vi "Main.vi"(8 "error in":errorcluster, 11 "New Worker in":refnum<class "Manager Worker.lvclass">) -> (0 "error out":errorcluster, 3 "New Worker out":refnum<class "Manager Worker.lvclass">)   [LabVIEW 2018, in "Manager Worker.lvclass"]
doc: "The Queued Message Handler of a Worker."
uses:
  Manager Worker.lvclass
  D:/Program Files (x86)/National Instruments/LabVIEW 2018/vi.lib/addons/_Workers/Library/Classes/Worker/Worker.lvclass
  Manager Worker.lvclass/Manager Worker.ctl
  <vilib>/addons/_Workers/Library/Classes/Worker/Worker.lvclass/Worker.ctl
  Initialization Data.ctl
  ChartView Worker/ChartView Worker.lvclass
  Config Worker/Config Worker.lvclass
  User Worker/User Worker.lvclass
  Comm Worker/Comm Worker.lvclass
  <vilib>/addons/_Workers/Library/Classes/Message/Enqueue Message to Queue.vi
  <vilib>/addons/_Workers/Library/Classes/Worker/Worker.lvclass
  <vilib>/addons/_Workers/Library/Classes/Message/Message.lvclass
  D:/Program Files (x86)/National Instruments/LabVIEW 2018/vi.lib/addons/_Workers/Library/Classes/Workers Object/Workers Object.lvclass
panel:
  in  "ButtonMenu":enum32{"ChartView", "Config", "User"}(radio)
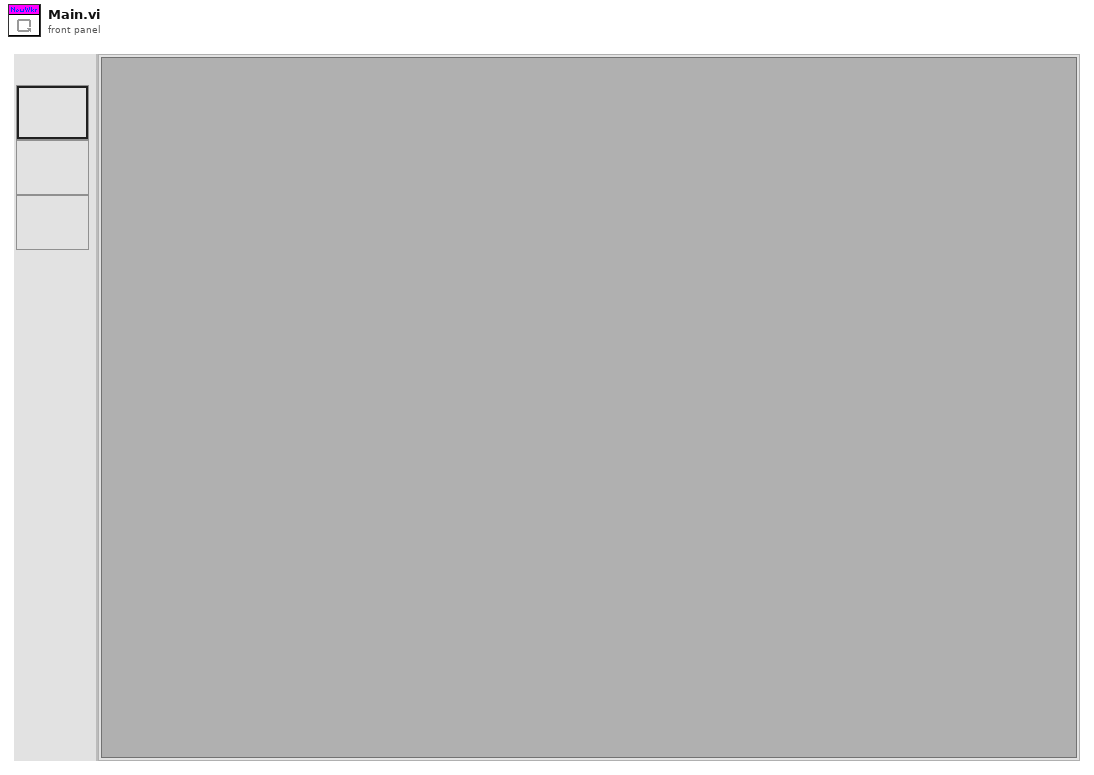
[diagram p1: front panel]
types:
  T1 = typedef "Manager Worker.lvclass/Initialization Data.ctl" = cluster{"String":string}
  T2 = typedef "Workers.lvlib/Case Label.ctl" = string
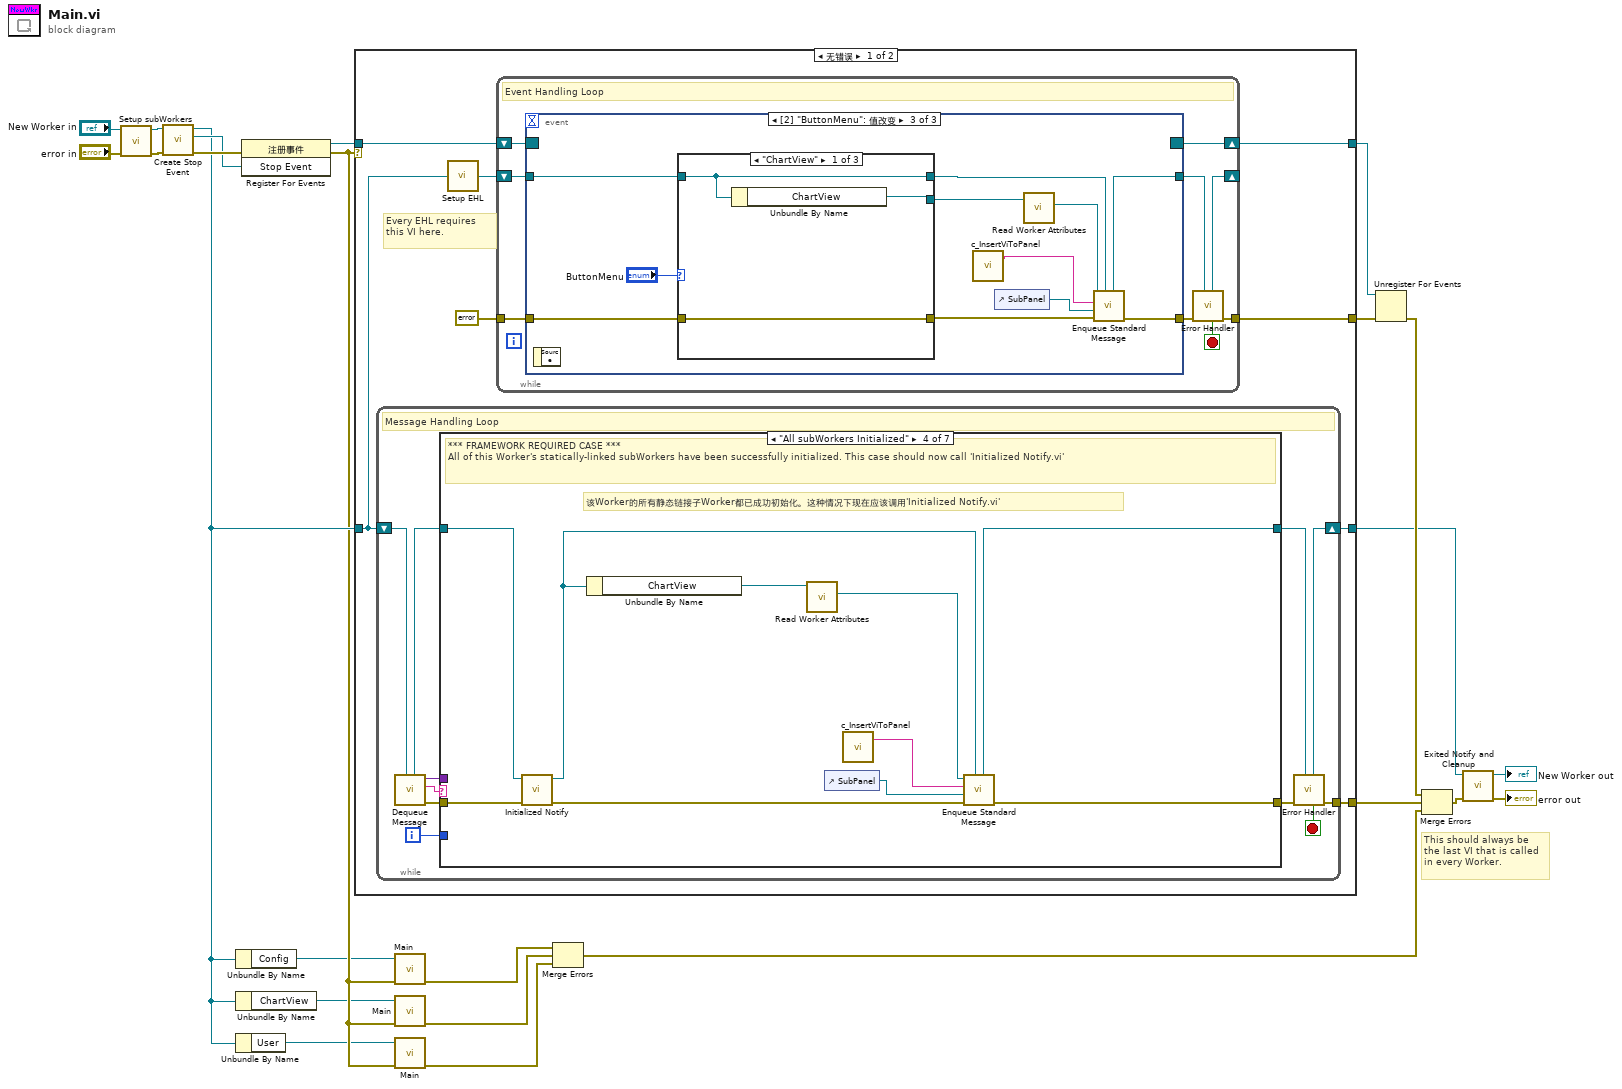
[diagram p0: block diagram]
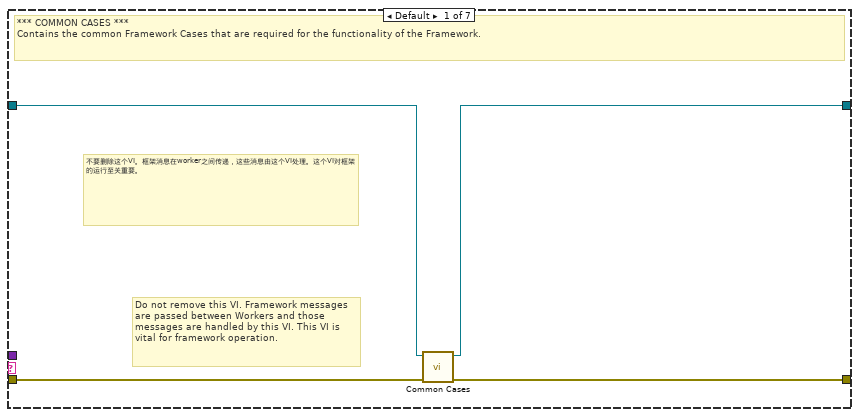
[diagram p2: hidden frame]
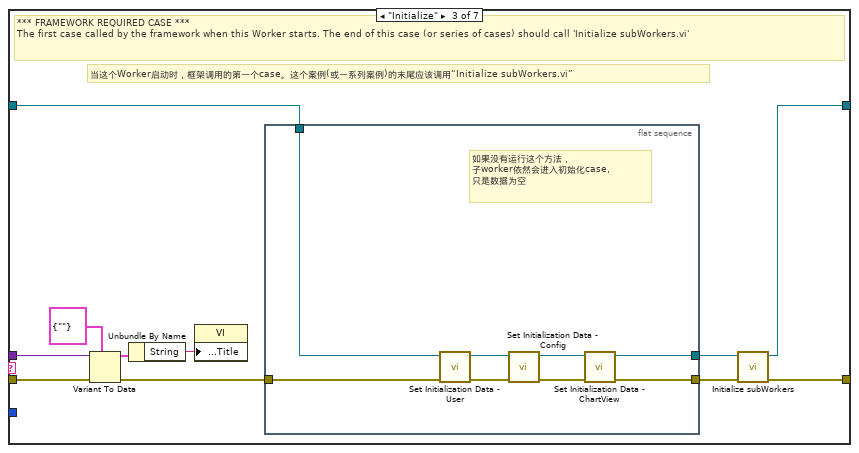
[diagram p4: hidden frame]
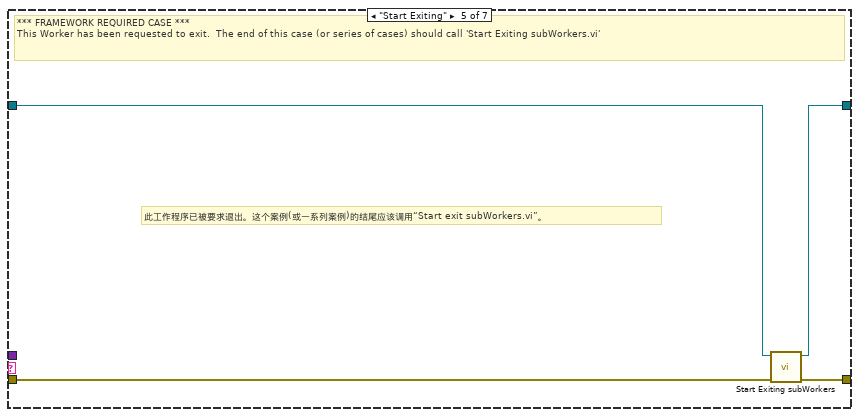
[diagram p5: hidden frame]
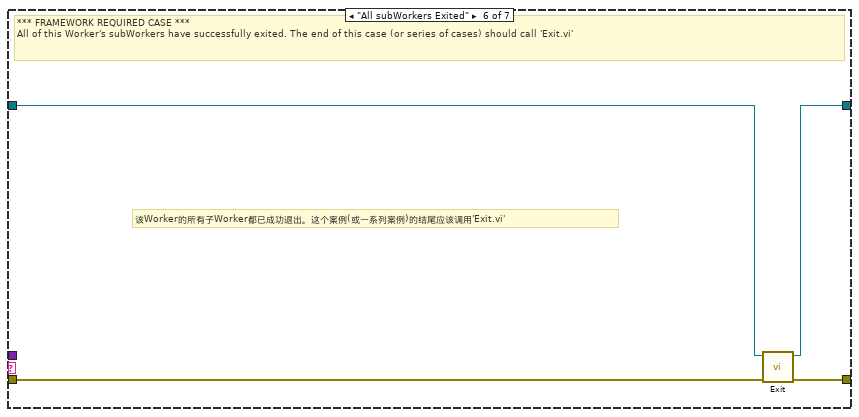
[diagram p6: hidden frame]
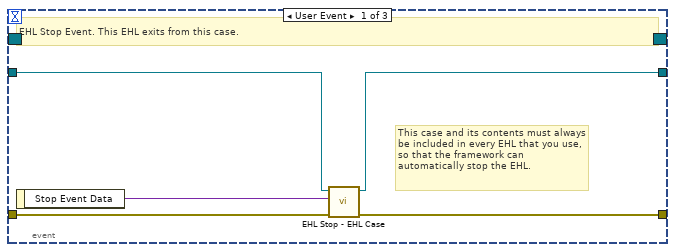
[diagram p8: hidden frame]
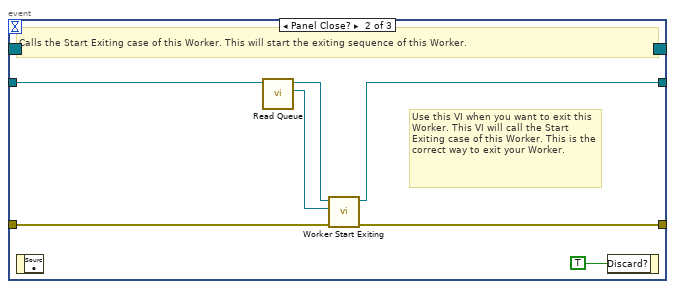
[diagram p9: hidden frame]
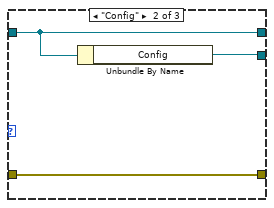
[diagram p10: hidden frame]
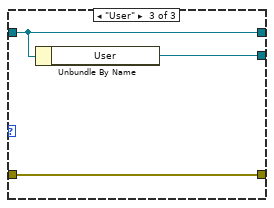
[diagram p11: hidden frame]
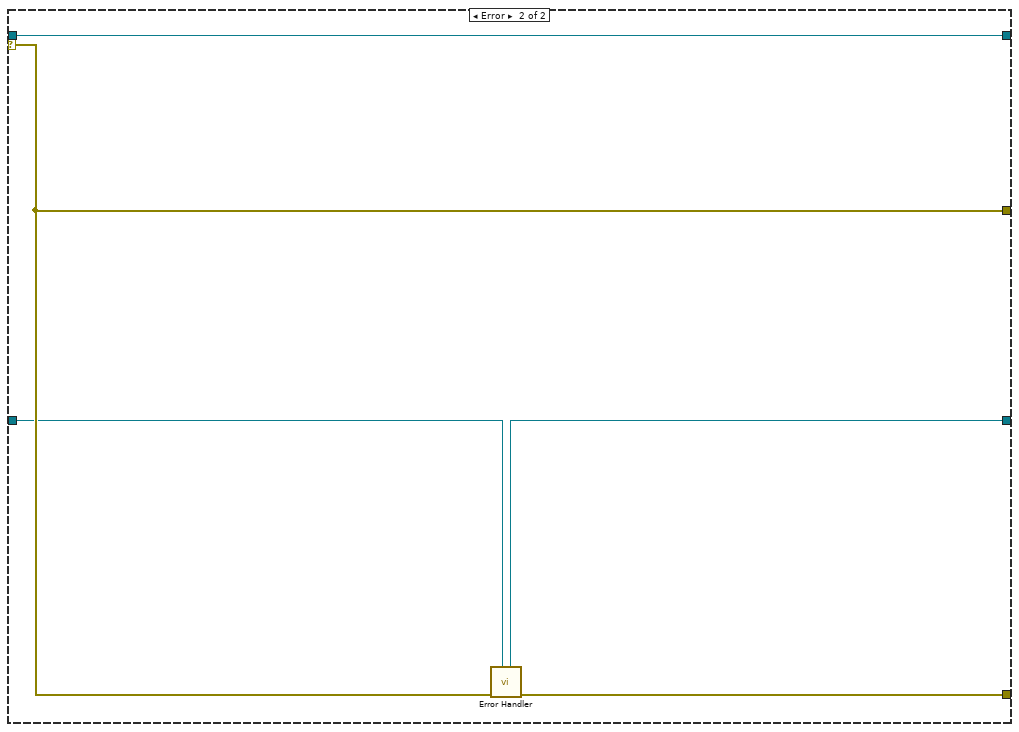
[diagram p12: hidden frame]
diagram:
  # "This should always be the last VI that is called in every Worker."
  n1 = call "Setup subWorkers.vi"("error in"="error in", "Manager Worker in"="New Worker in") -> ("error out"=w10:errorcluster, "Manager Worker out"=w8:refnum<class "Manager Worker.lvclass">)  [unwired: 8 in]
  n2 = call-dynamic "Create Stop Event.vi"("error in"=w10, "Worker"=w8) -> ("error out"=w19:errorcluster, "Stop Event"=w16:refnum<user-event>, "Worker out"=w13:refnum<class "Manager Worker.lvclass">)  [unwired: 7 in]
  n3 = Unbundle By Name(w13) -> ("Config"=w5:refnum<class "Config Worker.lvclass">)
  n4 = Unbundle By Name(w13) -> ("ChartView"=w3:refnum<class "ChartView Worker.lvclass">)
  n5 = Unbundle By Name(w13) -> ("User"=w1:refnum<class "User Worker.lvclass">)
  n6 = register-events(error in=w19, w16) -> (reference out=w18:refnum<event-registration>, error out=w11:errorcluster)  [unwired: 1 in]
  n7 = case shown="无错误" w11 {
    tunnel: w13 -> [w27 w131]
    tunnel: [w25 w132] -> w17
    tunnel: w18 -> [w32 w133]
    tunnel: [w29 w134] -> w23
    tunnel: [w31 w133] -> w22
    tunnel: [w26 w130] -> w20
    selector: w11 -> [_ w134]
    frame No Error {
      # "Every EHL requires\nthis VI here."
      n8 = while {
        shift-right: [w41] -> w26
        shift-left: w27 -> [w43]
        tunnel: [w42] -> w25
        i -> [w33]
        stop <- w34 stop-if-true
        # "Message Handling Loop"
        n9 = call-dynamic "Dequeue Message.vi"("Worker"=w43) -> ("error out"=w40:errorcluster, "Case out"=w35:string, "Data out"=w36:variant, "Worker out"=w38:refnum<class "Manager Worker.lvclass">)  [unwired: 6 in, 1 out]
        n10 = case "Worker MHL Case Structure (DO NOT CHANGE LABEL NAME)" shown="\"All subWorkers Initialized\"" w35 {
          tunnel: w40 -> [w47 w48 w58 w77 w79 w86 w87]
          tunnel: [w46 w48 w60 w75 w82 w85 w87] -> w39
          tunnel: w38 -> [w45 w49 w57 w78 w80 w84 w88]
          tunnel: [w44 w49 w59 w74 w81 w83 w88] -> w37
          tunnel: w36 -> [_ _ w56 _ _ _ _]
          tunnel: w33 -> [_ _ _ _ _ _ _]
          frame Default {
            # "不要删除这个VI。框架消息在worker之间传递，这些消息由这个VI处理。这个VI对框架的运行至关重要。"
            # "Do not remove this VI. Framework messages are passed between Workers and those messages are handled by this VI. This VI is vital for framework operation."
            # "*** COMMON CASES ***\nContains the common Framework Cases that are required for the functionality of the Framework."
            n11 = call-dynamic "Common Cases.vi"("error in"=w47, "Worker in"=w45) -> ("error out"=w46:errorcluster, "Worker out"=w44:refnum<class "Manager Worker.lvclass">)  [unwired: 8 in]
          }
          frame "------ FRAMEWORK REQUIRED CASES ------" {
            # "\"All subWorkers Exited\""
            # "\"Start Exiting\""
            # "\"All subWorkers Initialized\""
            # "\"Initialize\""
            # "启动机制。\n启动后会进入\"Initialize\" 分支，然后初始化下一层work.\n如果没有下一层work，则很快进入\"All subWorkers Initialized\" 分支。\n如果有下一层分支，则一层层的向下层初始化。然后又最底层的worker一层层向上发送 \"All subWorkers Initialized\" ，发送初始化完成通知。\n\n退出机制\n上层Worker进入\"Start Exiting\" 分支，向下一层发送 start Exiting Subworker。\n如果~~~\n如果有~~~\n与启动机制类似。"
            # "Start of Framework Required Cases"
          }
          frame "Initialize" {
            # "当这个Worker启动时，框架调用的第一个case。这个案例(或一系列案例)的末尾应该调用“Initialize subWorkers.vi”"
            # "*** FRAMEWORK REQUIRED CASE ***\nThe first case called by the framework when this Worker starts. The end of this case (or series of cases) should call 'Initialize subWorkers.vi'"
            n12 = Variant To Data(error in=w58, type=T1 {"String"=""} ("Initialization Data"), Variant=w56) -> (data=w54:T1, error out=w52:errorcluster)
            n13 = Unbundle By Name(w54) -> ("String"=w50:string)
            n14 = property class="VI"("Front Panel.Title"=w50) -> ()  [unwired: 2 in, 2 out]
            n15 = flat-sequence {
              tunnel: w57 -> [w68]
              tunnel: [w62] -> w53
              tunnel: w52 -> [w67]
              tunnel: [w61] -> w51
              frame #0 {
                # "如果没有运行这个方法，\n子worker依然会进入初始化case,\n只是数据为空"
                n16 = call "Set Initialization Data - User.vi"("error in"=w67, "Manager Worker in"=w68) -> ("error out"=w65:errorcluster, "Manager Worker out"=w66:refnum<class "Manager Worker.lvclass">)  [unwired: 8 in]
                n17 = call "Set Initialization Data - Config.vi"("error in"=w65, "Manager Worker in"=w66) -> ("error out"=w63:errorcluster, "Manager Worker out"=w64:refnum<class "Manager Worker.lvclass">)  [unwired: 8 in]
                n18 = call "Set Initialization Data - ChartView.vi"("error in"=w63, "Manager Worker in"=w64) -> ("error out"=w61:errorcluster, "Manager Worker out"=w62:refnum<class "Manager Worker.lvclass">)  [unwired: 8 in]
              }
            }
            n19 = call-dynamic "Initialize subWorkers.vi"("error in"=w51, "Worker"=w53) -> ("error out"=w60:errorcluster, "dup Worker out"=w59:refnum<class "Manager Worker.lvclass">)  [unwired: 8 in]
          }
          frame "All subWorkers Initialized" {
            # "该Worker的所有静态链接子Worker都已成功初始化。这种情况下现在应该调用'Initialized Notify.vi'"
            # "*** FRAMEWORK REQUIRED CASE ***\nAll of this Worker's statically-linked subWorkers have been successfully initialized. This case should now call 'Initialized Notify.vi'"
            n20 = call-dynamic "Initialized Notify.vi"("error in"=w77, "Worker"=w78) -> ("error out"=w76:errorcluster, "dup Worker out"=w72:refnum<class "Manager Worker.lvclass">)  [unwired: 8 in]
            n21 = Unbundle By Name(w72) -> ("ChartView"=w71:refnum<class "ChartView Worker.lvclass">)
            n22 = call-poly <vilib>:"Read Worker Attributes.vi"("Worker"=w71) -> ("Message Queue out"=w70:refnum<class "Message Queue.lvclass">)  [unwired: 9 in, 1 out]
            n23 = control-ref of="SubPanel"() -> (w69:refnum<vi>)
            n24 = call "c_InsertViToPanel.vi"() -> ("Case Label"=w73:T2)  [unwired: 1 in]
            n25 = call-poly <vilib>:"Enqueue Standard Message.vi"("Worker"=w72, "error in"=w76, "Data"=w69, "Case Label"=w73, "Message Queue"=w70) -> ("error out"=w75:errorcluster, "dup Worker out"=w74:refnum<class "Manager Worker.lvclass">)  [unwired: 4 in, 1 out]
          }
          frame "Start Exiting" {
            # "此工作程序已被要求退出。这个案例(或一系列案例)的结尾应该调用“Start exit subWorkers.vi”。"
            # "*** FRAMEWORK REQUIRED CASE ***\nThis Worker has been requested to exit.  The end of this case (or series of cases) should call 'Start Exiting subWorkers.vi'"
            n26 = call-dynamic "Start Exiting subWorkers.vi"("error_in"=w79, "Worker"=w80) -> ("error out"=w82:errorcluster, "dup Worker out"=w81:refnum<class "Manager Worker.lvclass">)  [unwired: 8 in]
          }
          frame "All subWorkers Exited" {
            # "该Worker的所有子Worker都已成功退出。这个案例(或一系列案例)的结尾应该调用'Exit.vi'"
            # "*** FRAMEWORK REQUIRED CASE ***\nAll of this Worker's subWorkers have successfully exited. The end of this case (or series of cases) should call 'Exit.vi'"
            n27 = call-dynamic "Exit.vi"("error_in"=w86, "Worker"=w84) -> ("error out"=w85:errorcluster, "dup Worker out"=w83:refnum<class "Manager Worker.lvclass">)  [unwired: 8 in]
          }
          frame "-----------------------------------------------" {
            # "End of Framework Required Cases"
          }
        }
        n28 = call-dynamic "Error Handler.vi"("Worker"=w37, "error_in"=w39) -> ("error out"=w42:errorcluster, "Stop Loop"=w34:bool, "Worker out"=w41:refnum<class "Manager Worker.lvclass">)  [unwired: 7 in]
      }
      n29 = call-dynamic "Setup EHL.vi"("Worker"=w27) -> ("Worker out"=w28:refnum<class "Manager Worker.lvclass">)  [unwired: 14 in]
      n30 = while "Event Handling Loop" {
        shift-right: [w97] -> w31
        shift-left: w32 -> [w96]
        tunnel: [w92] -> w29
        tunnel: errorcluster {"status"=FALSE, "code"=0, "source"=""} ("error constant") -> [w94]
        shift-right: [w90] -> _
        shift-left: w28 -> [w95]
        stop <- w89 stop-if-true
        # "Event Handling Loop"
        n31 = event shown="[2] \"ButtonMenu\": 值改变" {
          selector: w96 -> [_ _ _]
          dyn-events: [_ _ _] -> w97
          timeout: _ -> [_ _ _]
          tunnel: [w101 w108 w116] -> w93
          tunnel: w94 -> [w102 w107 w119]
          tunnel: w95 -> [w100 w106 w118]
          tunnel: [w99 w105 w115] -> w91
          event User Event {
            # "This case and its contents must always be included in every EHL that you use, so that the framework can automatically stop the EHL."
            # "EHL Stop Event. This EHL exits from this case."
            n32 = event-data() -> ("Stop Event Data"=w98:variant)  [unwired: 1 in]
            n33 = call <vilib>:"EHL Stop - EHL Case.vi"("error in"=w102, "Stop Event Data"=w98, "Worker"=w100) -> ("error out"=w101:errorcluster, "Worker out"=w99:refnum<class "Manager Worker.lvclass">)  [unwired: 7 in]
          }
          event Panel Close? {
            # "Use this VI when you want to exit this Worker. This VI will call the Start Exiting case of this Worker. This is the correct way to exit your Worker."
            # "Calls the Start Exiting case of this Worker. This will start the exiting sequence of this Worker."
            n34 = event-data() -> ()  [unwired: 1 in, 1 out]
            n35 = call <vilib>:"Read Queue.vi"("Worker"=w106) -> ("Message Queue out"=w103:refnum<class "Message Queue.lvclass">, "dup Worker out"=w104:refnum<class "Manager Worker.lvclass">)  [unwired: 9 in]
            n36 = call-dynamic "Worker Start Exiting.vi"("error_in"=w107, "Message Queue"=w103, "Worker"=w104) -> ("error out"=w108:errorcluster, "dup Worker out"=w105:refnum<class "Manager Worker.lvclass">)  [unwired: 7 in]
            n37 = event-data ("事件过滤节点")("Discard?"=TRUE) -> ()  [unwired: 1 in, 1 out]
          }
          event "ButtonMenu": Value Change {
            n38 = event-data() -> ()  [unwired: 1 in, 1 out]
            n39 = case shown="\"ChartView\"" "ButtonMenu" {
              tunnel: w119 -> [w123 w126 w129]
              tunnel: [w123 w126 w129] -> w117
              tunnel: [w122 w125 w127] -> w112
              tunnel: w118 -> [w122 w125 w127]
              tunnel: [w121 w124 w128] -> w113
              frame "ChartView" {
                n40 = Unbundle By Name(w122) -> ("ChartView"=w121:refnum<class "ChartView Worker.lvclass">)
              }
              frame "Config" {
                n41 = Unbundle By Name(w125) -> ("Config"=w124:refnum<class "Config Worker.lvclass">)
              }
              frame "User" {
                n42 = Unbundle By Name(w127) -> ("User"=w128:refnum<class "User Worker.lvclass">)
              }
            }
            n43 = call "c_InsertViToPanel.vi"() -> ("Case Label"=w110:T2)  [unwired: 1 in]
            n44 = control-ref of="SubPanel"() -> (w111:refnum<vi>)
            n45 = call-poly <vilib>:"Read Worker Attributes.vi"("Worker"=w113) -> ("Message Queue out"=w114:refnum<class "Message Queue.lvclass">)  [unwired: 9 in, 1 out]
            n46 = call-poly <vilib>:"Enqueue Standard Message.vi"("Worker"=w112, "error in"=w117, "Data"=w111, "Case Label"=w110, "Message Queue"=w114) -> ("error out"=w116:errorcluster, "dup Worker out"=w115:refnum<class "Manager Worker.lvclass">)  [unwired: 4 in, 1 out]
          }
        }
        n47 = call-dynamic "Error Handler.vi"("Worker"=w91, "error_in"=w93) -> ("error out"=w92:errorcluster, "Stop Loop"=w89:bool, "Worker out"=w90:refnum<class "Manager Worker.lvclass">)  [unwired: 7 in]
      }
    }
    frame Error {
      n48 = call-dynamic "Error Handler.vi"("Worker"=w131, "error_in"=w134) -> ("error out"=w132:errorcluster, "Worker out"=w130:refnum<class "Manager Worker.lvclass">)  [unwired: 7 in, 1 out]
    }
  }
  n49 = call-dynamic "Main.vi"("error in"=w11, "Config Worker in"=w5) -> ("error out"=w6:errorcluster)  [unwired: 8 in, 1 out]
  n50 = call-dynamic "Main.vi"("error in"=w11, "ChartView Worker in"=w3) -> ("error out"=w4:errorcluster)  [unwired: 8 in, 1 out]
  n51 = call-dynamic "Main.vi"("error in"=w11, "User Worker in"=w1) -> ("error out"=w2:errorcluster)  [unwired: 8 in, 1 out]
  n52 = Merge Errors(w6, w4, w2) -> (w7:errorcluster)
  n53 = Unregister For Events(event registration refnum=w22, error in=w23) -> (error out=w24:errorcluster)
  n54 = Merge Errors ("合并错误")(w24, w17, w7) -> (w21:errorcluster)
  n55 = call-dynamic "Exited Notify and Cleanup.vi"("error_in"=w21, "Worker"=w20) -> ("error out"=→"error out":errorcluster, "dup Worker out"=→"New Worker out":refnum<class "Manager Worker.lvclass">)  [unwired: 8 in]
